vi "Create Table.vi"(1 "Table Name":string) -> (0 "resulting string":string)   [LabVIEW 2020]
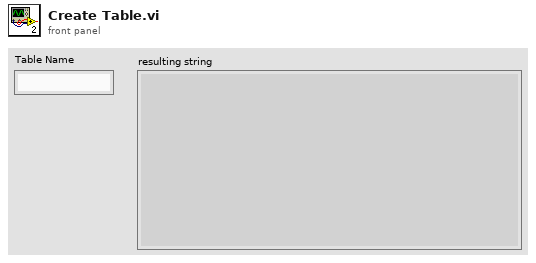
[diagram p1: front panel]
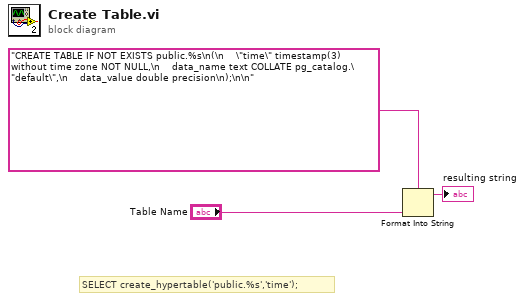
[diagram p0: block diagram]
diagram:
  # "SELECT create_hypertable('public.%s','time');"
  n1 = Format Into String(format string="CREATE TABLE IF NOT EXISTS public.%s\n(\n    \"time\" timestamp(3) without time zone NOT NULL,\n    data_name text COLLATE pg_catalog.\"default\",\n    data_value double precision\n);\n\n", "Table Name") -> (resulting string=→"resulting string":string)  [unwired: 2 in, 1 out]
